vi "myRIO_BRig_Host_comm_getData_1D_u16.vi"(11 "input_fileName":string) -> (2 "output_data_1D":u16[](array[numeric]), 3 "output_I_data":bool)   [LabVIEW 2014]
uses:
  <vilib>/Utility/file.llb/Read From Spreadsheet File (I64).vi
panel:
  out "error out":errorcluster
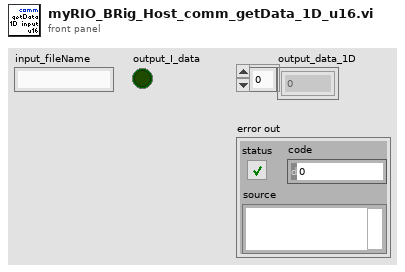
[diagram p1: front panel]
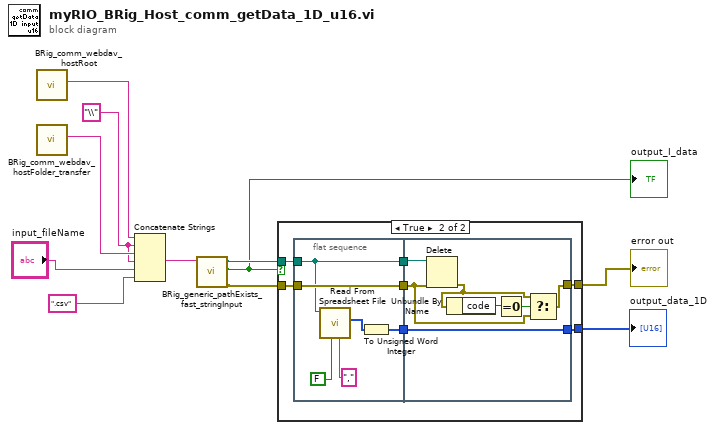
[diagram p0: block diagram]
diagram:
  w6 = "\\" ("string")
  n1 = call "BRig_comm_webdav_hostRoot.vi"() -> ("output_hostRoot"=w9:string)  [unwired: 11 in]
  n2 = call "BRig_comm_webdav_hostFolder_transfer.vi"() -> ("output_HostFolder"=w10:string)  [unwired: 11 in]
  n3 = Concatenate Strings(w9, w6, w10, w6, "input_fileName", ".csv" ("string")) -> (w5:string)
  n4 = call "BRig_generic_pathExists_fast_stringInput.vi"("input_filePath"=w5) -> ("output_error"=w2:errorcluster, "output_Iexist"=w3:bool, "output_filePath"=w4:path)  [unwired: 8 in]
  "output_I_data" <- w3
  n5 = case shown="True" w3 {
    tunnel: w4 -> [_ w19]
    tunnel: w2 -> [w12 w16]
    tunnel: [_ w14] -> w11
    tunnel: [w12 w13] -> w1
    frame False {
    }
    frame True {
      n6 = flat-sequence {
        tunnel: w19 -> [w23]
        tunnel: [w23] -> w18
        tunnel: w16 -> [w25]
        tunnel: [w25] -> w17
        tunnel: [w21] -> w15
        tunnel: w18 -> [w31]
        tunnel: w17 -> [w26]
        tunnel: [w32] -> w14
        tunnel: w15 -> [w32]
        tunnel: [w27] -> w13
        frame #0 {
          n7 = call-poly <vilib>:"Read From Spreadsheet File.vi"("delimiter (\\t)"="," ("delimiter (\\t)"), "transpose (no:F)"=FALSE, "file path (dialog if empty)"=w23) -> ("first row"=w20:i64[])  [unwired: 4 in, 4 out]
          n8 = To Unsigned Word Integer(number=w20) -> (unsigned 16bit integer=w21:u16[])
        }
        frame #1 {
          n9 = Delete(path (use dialog)=w31, error in=w26) -> (error out=w28:errorcluster)  [unwired: 3 in, 2 out]
          n10 = Unbundle By Name(w28) -> ("code"=w30:i32)
          n11 = Equal To 0?(x=w30) -> (x = 0?=w29:bool)
          n12 = Select(t=w28, s=w29, f=w26) -> (s? t:f=w27:errorcluster)
        }
      }
    }
  }
  "output_data_1D" <- w11
  "error out" <- w1
